vi "MotorMain.vi"() -> ()   [LabVIEW 2011]
uses:
  Modules/PIMotorController/PI_Axis_list.ctl
  Modules/PIMotorController/PI_Axis.ctl
  Main/Motors/MotorConfigType.ctl
  Main/Motors/MotorPosType.ctl
  Main/Typedefs/XYf.ctl
  Main/Motors/MotorPosFlagsType.ctl
panel:
  out "Conn. \nAxes 2":string[](array[string])
  out "Conn. Axes":string[](array[string])
  out "All conn. axes":string[](array[string])
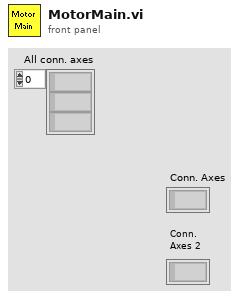
[diagram p1: front panel]
types:
  T1 = typedef "PI_Axis_list.ctl" = cluster{"Piezo X":T2, "Piezo Y":T2, "Piezo Z":T2, "Magnet Z":T2, "Magnet Rotation":T2, "Objective X":T2, "Objective Y":T2}
  T2 = typedef "PI_Axis.ctl" = cluster{"System #":i32, "Axis ID":string, "Multiplier":dbl}
  T3 = typedef "MotorConfigType.ctl" = cluster{"Offset":T4, "Maximum pos":T4, "Min limited?":T6, "Max limited?":T6, "Has velocity support":T6, "Default velocity":T4}
  T4 = typedef "MotorPosType.ctl" = cluster{"Magnet Z":dbl, "Magnet rotation":dbl, "Camera":T5, "Piezo XY":T5, "Piezo Z":dbl, "Coil XY":T5}
  T5 = typedef "XYf.ctl" = cluster{"X":sgl, "Y":sgl}
  T6 = typedef "MotorPosFlagsType.ctl" = cluster{"Magnet Z":bool, "Magnet rotation":bool, "Camera":cluster{"X":bool, "Y":bool}, "Piezo XY":cluster{"X":bool, "Y":bool}, "Piezo Z":bool, "Coil XY":cluster{"X":bool, "Y":bool}}
  T7 = typedef "GCS_Interface.ctl" = cluster{"MOV":refnum<vi>, "VEL":refnum<vi>, "VEL?":refnum<vi>, "POS?":refnum<vi>, "TMX?":refnum<vi>, "#7 (Ready?)":refnum<vi>, "FPL":refnum<vi>, "FNL":refnum<vi>}
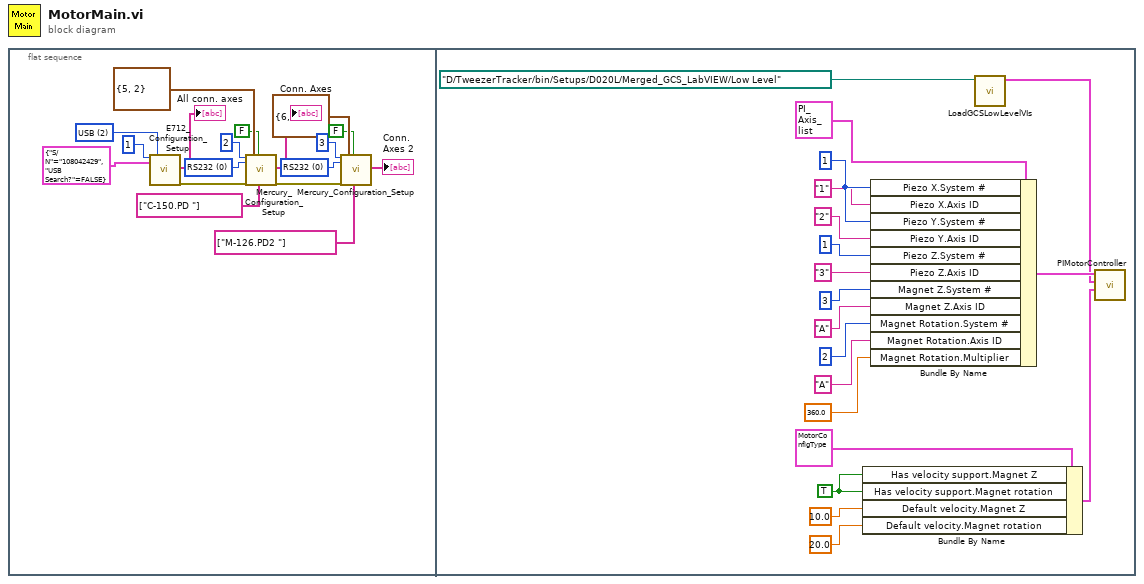
[diagram p0: block diagram]
diagram:
  n1 = flat-sequence {
    frame #0 {
      w11 = u16 0 items=["RS232", "RS232 DaisyChain", "USB", "USB_DaisyChain"] ("Interface")
      w13 = u16 0 items=["RS232", "RS232 DaisyChain", "USB", "USB_DaisyChain"] ("Interface")
      w17 = u16 2 items=["RS232", "TCP/IP", "USB"] ("Interface")
      n2 = call "E712_Configuration_Setup.vi"("System no."=1, "USB settings"=cluster{"S/N":string, "USB Search?":bool} {"S/N"="108042429", "USB Search?"=FALSE}, "Interface"=w17) -> ("All conn. axes"=→"All conn. axes":string[], "error out"=w14:errorcluster)  [unwired: 12 in, 3 out]
      n3 = call "Mercury_Configuration_Setup.vi"("System no."=2, "error in"=w14, "RS232 settings"=cluster{"Portnumber":i32, "Baudrate":i32} {"Portnumber"=5, "Baudrate"=2}, "Use dialog to define\nconnected stages?"=FALSE ("Use dialog to define\nconnected stages?"), "Stage names input"=string[] ["C-150.PD "], "Limit switch selection"=w13) -> ("Conn. \nAxis"=→"Conn. Axes":string[], "error out"=w8:errorcluster)  [unwired: 9 in, 3 out]
      n4 = call "Mercury_Configuration_Setup.vi"("System no."=3, "error in"=w8, "RS232 settings"=cluster{"Portnumber":i32, "Baudrate":i32} {"Portnumber"=6, "Baudrate"=2}, "Use dialog to define\nconnected stages?"=FALSE ("Use dialog to define\nconnected stages?"), "Stage names input"=string[] ["M-126.PD2 "], "Limit switch selection"=w11) -> ("Conn. \nAxis"=→"Conn. \nAxes 2":string[])  [unwired: 9 in, 4 out]
    }
    frame #1 {
      w30 = TRUE ("Has velocity support.Magnet Z")
      w36 = 1 ("Piezo X.System #")
      n5 = Bundle By Name(cluster=T3 {"Offset"={"Magnet Z"=0.0, "Magnet rotation"=0.0, "Camera"={"X"=0.0, "Y"=0.0}, "Piezo XY"={"X"=0.0, "Y"=0.0}, "Piezo Z"=0.0, "Coil XY"={"X"=0.0, "Y"=0.0}}, "Maximum pos"={"Magnet Z"=0.0, "Magnet rotation"=0.0, "Camera"={"X"=0.0, "Y"=0.0}, "Piezo XY"={"X"=0.0, "Y"=0.0}, "Piezo Z"=0.0, "Coil XY"={"X"=0.0, "Y"=0.0}}, "Min limited?"={"Magnet Z"=FALSE, "Magnet rotation"=FALSE, "Camera"={"X"=FALSE, "Y"=FALSE}, "Piezo XY"={"X"=FALSE, "Y"=FALSE}, "Piezo Z"=FALSE, "Coil XY"={"X"=FALSE, "Y"=FALSE}}, "Max limited?"={"Magnet Z"=FALSE, "Magnet rotation"=FALSE, "Camera"={"X"=FALSE, "Y"=FALSE}, "Piezo XY"={"X"=FALSE, "Y"=FALSE}, "Piezo Z"=FALSE, "Coil XY"={"X"=FALSE, "Y"=FALSE}}, "Has velocity support"={"Magnet Z"=TRUE, "Magnet rotation"=TRUE, "Camera"={"X"=FALSE, "Y"=FALSE}, "Piezo XY"={"X"=FALSE, "Y"=FALSE}, "Piezo Z"=FALSE, "Coil XY"={"X"=FALSE, "Y"=FALSE}}, "Default velocity"={"Magnet Z"=0.0, "Magnet rotation"=0.0, "Camera"={"X"=0.0, "Y"=0.0}, "Piezo XY"={"X"=0.0, "Y"=0.0}, "Piezo Z"=0.0, "Coil XY"={"X"=0.0, "Y"=0.0}}} ("MotorConfig"), "Has velocity support.Magnet Z"=w30, "Has velocity support.Magnet rotation"=w30, "Default velocity.Magnet Z"=10.0, "Default velocity.Magnet rotation"=20.0) -> (w19:T3)
      n6 = Bundle By Name(cluster=T1 {"Piezo X"={"System #"=0, "Axis ID"="", "Multiplier"=1.0}, "Piezo Y"={"System #"=0, "Axis ID"="", "Multiplier"=1.0}, "Piezo Z"={"System #"=0, "Axis ID"="", "Multiplier"=1.0}, "Magnet Z"={"System #"=0, "Axis ID"="", "Multiplier"=1.0}, "Magnet Rotation"={"System #"=0, "Axis ID"="", "Multiplier"=1.0}, "Objective X"={"System #"=0, "Axis ID"="", "Multiplier"=1.0}, "Objective Y"={"System #"=0, "Axis ID"="", "Multiplier"=1.0}} ("PI Axis config"), "Piezo X.System #"=w36, "Piezo X.Axis ID"="1", "Piezo Y.System #"=w36, "Piezo Y.Axis ID"="2", "Piezo Z.System #"=1, "Piezo Z.Axis ID"="3", "Magnet Z.System #"=3, "Magnet Z.Axis ID"="A", "Magnet Rotation.System #"=2, "Magnet Rotation.Axis ID"="A", "Magnet Rotation.Multiplier"=360.0) -> (w21:T1)
      n7 = call "LoadGCSLowLevelVIs.vi"("GCS Merged Drivers Low-Level Path"=path "D:/TweezerTracker/bin/Setups/D020L/Merged_GCS_LabVIEW/Low Level") -> ("PI GCS Function\nReferences"=w20:T7)  [unwired: 10 in]
      n8 = call "PIMotorController.vi"("MotorConfig"=w19, "PI GCS Function\nReferences"=w20, "PI Axis config"=w21) -> ()  [unwired: 9 in]
    }
  }
